vi "Inclinometer.vi"   [LabVIEW 2016]
uses:
  Scratch/FPGASerial/DataTypes/SerialSettings.ctl
  Common_FPGA_Timestamp/DataTypes/TimestampSettings.ctl
  Common_FPGA_Modbus/DataTypes/ModbusCRCSettings.ctl
  Common_FPGA_T7Inclinometer/DataTypes/T7InclinometerSettings.ctl
  Common_FPGA_HealthAndStatus/DataTypes/HealthAndStatusSettings.ctl
  Common_FPGA_HealthAndStatus/DataTypes/HealthAndStatusFIFOCopySettings.ctl
  Scratch/FPGASerial/FPGASerial.lvlib
  Common_FPGA_Timestamp/FPGATimestamp.lvlib
  Common_FPGA_T7Inclinometer/FPGAT7Inclinometer.lvlib
  Common_FPGA_Modbus/FPGAModbus.lvlib
  Common_FPGA_HealthAndStatus/FPGAHealthAndStatus.lvlib
types:
  T1 = typedef "FPGAHealthAndStatus.lvlib/HealthAndStatusFIFOCopySettings.ctl" = cluster{"InternalHealthAndStatusFIFO":refnum<k21>, "SourceHealthAndStatusFIFO":refnum<k21>}
  T2 = typedef "FPGAHealthAndStatus.lvlib/HealthAndStatusSettings.ctl" = cluster{"InternalHealthAndStatusFIFO":refnum<k21>, "HealthAndStatusQueryFIFO":refnum<k21>, "HealthAndStatusResponseFIFO":refnum<k21>, "HealthAndStatusMemory":refnum<k21>, "MemorySize":i32}
  T3 = typedef "FPGAT7Inclinometer.lvlib/T7InclinometerSettings.ctl" = cluster{"SerialTxFIFO":refnum<k21>, "SerialRxFIFO":refnum<k21>, "TimestampRegister":refnum<k21>, "DataFIFO":refnum<k21>, "CRCDataFIFO":refnum<k21>, "CRCCalculateFIFO":refnum<k21>, "CRCFIFO":refnum<k21>, "HealthAndStatusFIFO":refnum<k21>, "BaseHealthAndStatusAddress":u32}
  T4 = typedef "FPGAModbus.lvlib/ModbusCRCSettings.ctl" = cluster{"DataFIFO":refnum<k21>, "CalculateFIFO":refnum<k21>, "OutputFIFO":refnum<k21>}
  T5 = typedef "FPGATimestamp.lvlib/TimestampSettings.ctl" = cluster{"TimeRegister":refnum<k21>, "TimeSource":refnum<k21>, "IterationsPerMicrosecond":i16, "UpdateFIFO":refnum<k21>}
  T6 = typedef "FPGASerial.lvlib/SerialSettings.ctl" = cluster{"SerialPort":refnum<k21>, "TxFIFO":refnum<k21>, "RxFIFO":refnum<k21>}
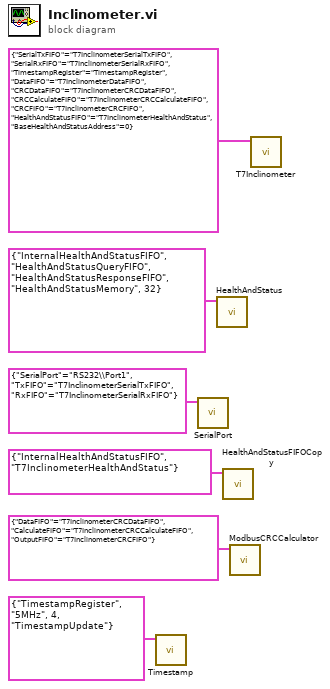
[diagram p0: block diagram]
diagram:
  n1 = call "Timestamp.vi"("TimestampSettings"=T5 {"TimeRegister"="TimestampRegister", "TimeSource"="5MHz", "IterationsPerMicrosecond"=4, "UpdateFIFO"="TimestampUpdate"}) -> ()  [unwired: 11 in]
  n2 = call "SerialPort.vi"("SerialSettings"=T6 {"SerialPort"="RS232\\Port1", "TxFIFO"="T7InclinometerSerialTxFIFO", "RxFIFO"="T7InclinometerSerialRxFIFO"}) -> ()  [unwired: 11 in]
  n3 = call "HealthAndStatus.vi"("HealthAndStatusSettings"=T2 {"InternalHealthAndStatusFIFO"="InternalHealthAndStatusFIFO", "HealthAndStatusQueryFIFO"="HealthAndStatusQueryFIFO", "HealthAndStatusResponseFIFO"="HealthAndStatusResponseFIFO", "HealthAndStatusMemory"="HealthAndStatusMemory", "MemorySize"=32}) -> ()  [unwired: 11 in]
  n4 = call "HealthAndStatusFIFOCopy.vi"("HealthAndStatusSettingsFIFOCopySettings"=T1 {"InternalHealthAndStatusFIFO"="InternalHealthAndStatusFIFO", "SourceHealthAndStatusFIFO"="T7InclinometerHealthAndStatus"}) -> ()  [unwired: 11 in]
  n5 = call "ModbusCRCCalculator.vi"("ModbusCRCSettings"=T4 {"DataFIFO"="T7InclinometerCRCDataFIFO", "CalculateFIFO"="T7InclinometerCRCCalculateFIFO", "OutputFIFO"="T7InclinometerCRCFIFO"}) -> ()  [unwired: 11 in]
  n6 = call "T7Inclinometer.vi"("T7InclinometerSettings"=T3 {"SerialTxFIFO"="T7InclinometerSerialTxFIFO", "SerialRxFIFO"="T7InclinometerSerialRxFIFO", "TimestampRegister"="TimestampRegister", "DataFIFO"="T7InclinometerDataFIFO", "CRCDataFIFO"="T7InclinometerCRCDataFIFO", "CRCCalculateFIFO"="T7InclinometerCRCCalculateFIFO", "CRCFIFO"="T7InclinometerCRCFIFO", "HealthAndStatusFIFO"="T7InclinometerHealthAndStatus", "BaseHealthAndStatusAddress"=0}) -> ()  [unwired: 11 in]
